vi "test.vi"() -> ()   [LabVIEW 2017]
uses:
  <vilib>/imath/engines/lvmath/Plug In/_Char/NIMS_CH_character datatype.ctl
  <vilib>/imath/engines/lvmath2/RunTimeEngine/Managers/WorkSpace/UID Generator.vi
  <vilib>/imath/engines/lvmath/Plug In/_Char/NIMS_CH_Character RV to String.vi
  <vilib>/imath/engines/lvmath2/RunTimeEngine/BuiltInFunctions/title/NIMS_title.vi
  <vilib>/imathl/engines/lvmath/Functions/Error Handling/Create Error.vi
  <vilib>/imath/engines/lvmath2/RunTimeEngine/BuiltInFunctions/xlimit/NIMS_xlimit.vi
  <vilib>/imath/engines/lvmath2/RunTimeEngine/BuiltInFunctions/ylimit/NIMS_ylimit.vi
  <vilib>/imath/engines/lvmath2/RunTimeEngine/BuiltInFunctions/hold/NIMS_hold(Enums).vi
  <vilib>/imath/engines/lvmath2/RunTimeEngine/IndexRead/NIMS M($,S).vi
  <instcachedir>/0/NIMS M($,S)_3E5749BBB62E49528D4765A77F1F6D98.lvgen/NIMS M($,S)_3E5749BBB62E49528D4765A77F1F6D98_002.vi
  <vilib>/imath/engines/lvmath2/RunTimeEngine/ErrorHandling/NIMS_Create Error From Enums.vi
  <vilib>/imath/engines/lvmath2/RunTimeEngine/BuiltInFunctions/plot/NIMS_plot(RM, RM, Str).vi
  <vilib>/imath/engines/lvmath2/RunTimeEngine/ErrorHandling/NIMS_Finalize Error.vi
  <vilib>/Utility/file.llb/Write Delimited Spreadsheet (DBL).vi
  <vilib>/vision/NI_Vision_Development_Module.lvlib
panel:
  out "robot  arrived":bool
  in  "SHOW TARGET POSITION":bool
  out "Image Out 4":T1(plugin-control)
  in  "see obstacle":bool
  out "Image Out 3":T1(plugin-control)
  in  "target array":dbl[][](array[numeric])
  out "target y position":sgl
  out "target x position":sgl
  out "robot y  position":sgl
  out "robot x position":sgl
  in  "Showing motion path":bool
  in  "robot array":dbl[][](array[numeric])
  out "robot is not in the picture":bool
  in  "check that robot is in the picture or not":bool
  out "Distance":sgl
  out "red":sgl[](array[numeric])
  out "target":sgl[](array[numeric])
  out "red Position":cluster{"x":sgl, "y":sgl}
  out "Image Out 2":T1(plugin-control)
  out "Blue Position":cluster{"x":sgl, "y":sgl}
  in  "Stop (F)":bool
  out "Image Out":T1(plugin-control)
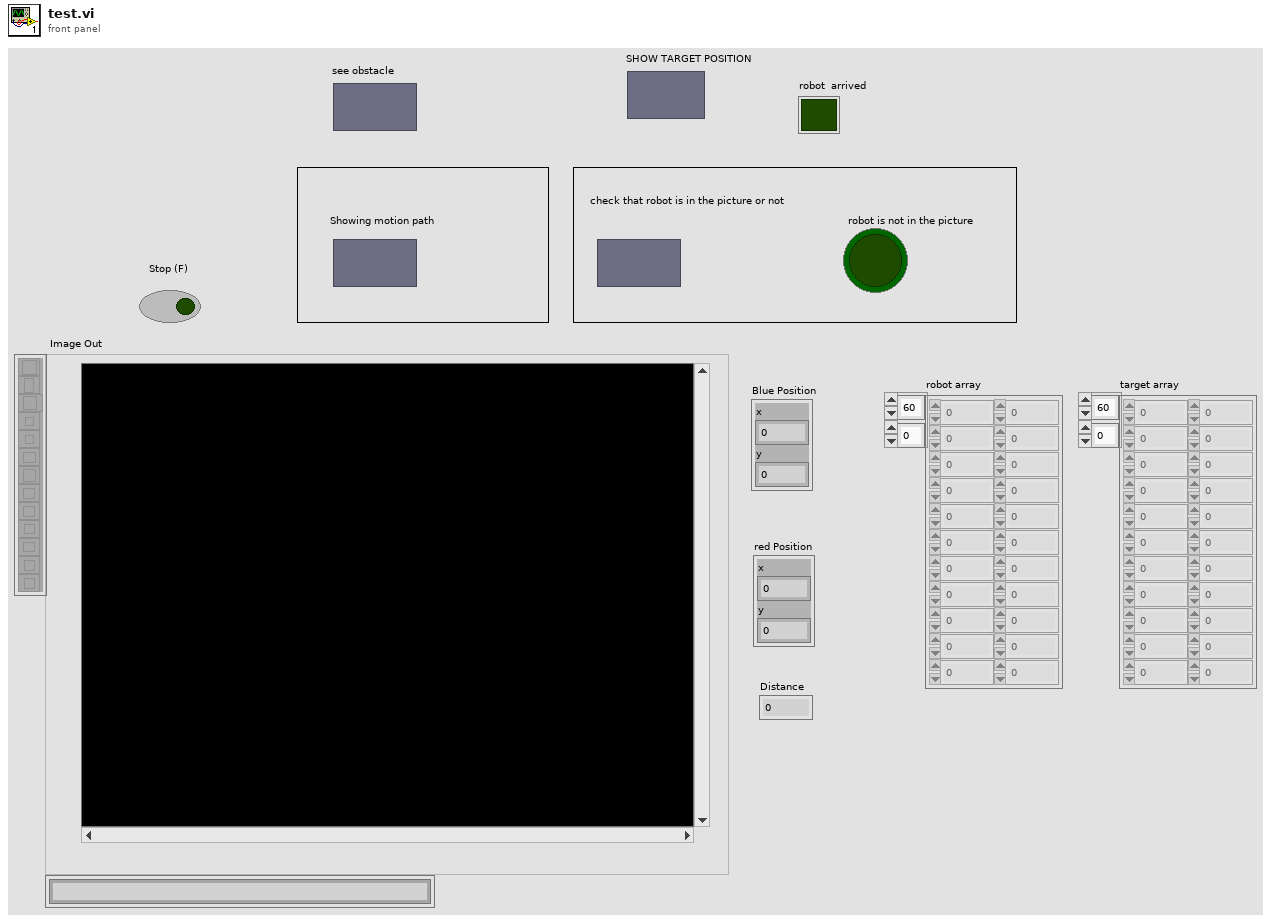
[diagram p1: front panel]
types:
  T1 = typedef "IMAQ Image.ctl" = refnum<image>
  T2 = typedef "Image Type" = u32
  T3 = typedef "NIMS_CH_character datatype.ctl" = cluster{"Numeric":u8}
  T4 = cluster{"Position":cluster{"x":sgl, "y":sgl}, "Angle":sgl, "Scale":sgl, "Score":sgl, "Bounding Box":cluster{"x":sgl, "y":sgl}[]}[]
  T5 = cluster{"Matches (Color Location 3)[0]":cluster{"Position":cluster{"x":sgl, "y":sgl}, "Angle":sgl, "Scale":sgl, "Score":sgl, "Bounding Box":cluster{"x":sgl, "y":sgl}[]}, "Matches (Color Location 3)[1]":cluster{"Position":cluster{"x":sgl, "y":sgl}, "Angle":sgl, "Scale":sgl, "Score":sgl, "Bounding Box":cluster{"x":sgl, "y":sgl}[]}, "Matches (Color Location 3)[2]":cluster{"Position":cluster{"x":sgl, "y":sgl}, "Angle":sgl, "Scale":sgl, "Score":sgl, "Bounding Box":cluster{"x":sgl, "y":sgl}[]}, "Matches (Color Location 3)[3]":cluster{"Position":cluster{"x":sgl, "y":sgl}, "Angle":sgl, "Scale":sgl, "Score":sgl, "Bounding Box":cluster{"x":sgl, "y":sgl}[]}, "Matches (Color Location 3)[4]":cluster{"Position":cluster{"x":sgl, "y":sgl}, "Angle":sgl, "Scale":sgl, "Score":sgl, "Bounding Box":cluster{"x":sgl, "y":sgl}[]}, "Matches (Color Location 3)[5]":cluster{"Position":cluster{"x":sgl, "y":sgl}, "Angle":sgl, "Scale":sgl, "Score":sgl, "Bounding Box":cluster{"x":sgl, "y":sgl}[]}, "Matches (Color Location 3)[6]":cluster{"Position":cluster{"x":sgl, "y":sgl}, "Angle":sgl, "Scale":sgl, "Score":sgl, "Bounding Box":cluster{"x":sgl, "y":sgl}[]}, "Matches (Color Location 3)[7]":cluster{"Position":cluster{"x":sgl, "y":sgl}, "Angle":sgl, "Scale":sgl, "Score":sgl, "Bounding Box":cluster{"x":sgl, "y":sgl}[]}, "Matches (Color Location 3)[8]":cluster{"Position":cluster{"x":sgl, "y":sgl}, "Angle":sgl, "Scale":sgl, "Score":sgl, "Bounding Box":cluster{"x":sgl, "y":sgl}[]}}
  T6 = cluster{"Bounding Box[0]":cluster{"x":sgl, "y":sgl}, "Bounding Box[1]":cluster{"x":sgl, "y":sgl}, "Bounding Box[2]":cluster{"x":sgl, "y":sgl}, "Bounding Box[3]":cluster{"x":sgl, "y":sgl}, "Bounding Box[4]":cluster{"x":sgl, "y":sgl}, "Bounding Box[5]":cluster{"x":sgl, "y":sgl}, "Bounding Box[6]":cluster{"x":sgl, "y":sgl}, "Bounding Box[7]":cluster{"x":sgl, "y":sgl}, "Bounding Box[8]":cluster{"x":sgl, "y":sgl}}
  T7 = cluster{"[0]":sgl, "[1]":sgl, "[2]":sgl, "[3]":sgl}
  T8 = cluster{"Matches (Color Location 1)[0]":cluster{"Position":cluster{"x":sgl, "y":sgl}, "Angle":sgl, "Scale":sgl, "Score":sgl, "Bounding Box":cluster{"x":sgl, "y":sgl}[]}, "Matches (Color Location 1)[1]":cluster{"Position":cluster{"x":sgl, "y":sgl}, "Angle":sgl, "Scale":sgl, "Score":sgl, "Bounding Box":cluster{"x":sgl, "y":sgl}[]}, "Matches (Color Location 1)[2]":cluster{"Position":cluster{"x":sgl, "y":sgl}, "Angle":sgl, "Scale":sgl, "Score":sgl, "Bounding Box":cluster{"x":sgl, "y":sgl}[]}, "Matches (Color Location 1)[3]":cluster{"Position":cluster{"x":sgl, "y":sgl}, "Angle":sgl, "Scale":sgl, "Score":sgl, "Bounding Box":cluster{"x":sgl, "y":sgl}[]}, "Matches (Color Location 1)[4]":cluster{"Position":cluster{"x":sgl, "y":sgl}, "Angle":sgl, "Scale":sgl, "Score":sgl, "Bounding Box":cluster{"x":sgl, "y":sgl}[]}, "Matches (Color Location 1)[5]":cluster{"Position":cluster{"x":sgl, "y":sgl}, "Angle":sgl, "Scale":sgl, "Score":sgl, "Bounding Box":cluster{"x":sgl, "y":sgl}[]}, "Matches (Color Location 1)[6]":cluster{"Position":cluster{"x":sgl, "y":sgl}, "Angle":sgl, "Scale":sgl, "Score":sgl, "Bounding Box":cluster{"x":sgl, "y":sgl}[]}, "Matches (Color Location 1)[7]":cluster{"Position":cluster{"x":sgl, "y":sgl}, "Angle":sgl, "Scale":sgl, "Score":sgl, "Bounding Box":cluster{"x":sgl, "y":sgl}[]}, "Matches (Color Location 1)[8]":cluster{"Position":cluster{"x":sgl, "y":sgl}, "Angle":sgl, "Scale":sgl, "Score":sgl, "Bounding Box":cluster{"x":sgl, "y":sgl}[]}}
  T9 = cluster{"Matches (Color Location 2)[0]":cluster{"Position":cluster{"x":sgl, "y":sgl}, "Angle":sgl, "Scale":sgl, "Score":sgl, "Bounding Box":cluster{"x":sgl, "y":sgl}[]}, "Matches (Color Location 2)[1]":cluster{"Position":cluster{"x":sgl, "y":sgl}, "Angle":sgl, "Scale":sgl, "Score":sgl, "Bounding Box":cluster{"x":sgl, "y":sgl}[]}, "Matches (Color Location 2)[2]":cluster{"Position":cluster{"x":sgl, "y":sgl}, "Angle":sgl, "Scale":sgl, "Score":sgl, "Bounding Box":cluster{"x":sgl, "y":sgl}[]}, "Matches (Color Location 2)[3]":cluster{"Position":cluster{"x":sgl, "y":sgl}, "Angle":sgl, "Scale":sgl, "Score":sgl, "Bounding Box":cluster{"x":sgl, "y":sgl}[]}, "Matches (Color Location 2)[4]":cluster{"Position":cluster{"x":sgl, "y":sgl}, "Angle":sgl, "Scale":sgl, "Score":sgl, "Bounding Box":cluster{"x":sgl, "y":sgl}[]}, "Matches (Color Location 2)[5]":cluster{"Position":cluster{"x":sgl, "y":sgl}, "Angle":sgl, "Scale":sgl, "Score":sgl, "Bounding Box":cluster{"x":sgl, "y":sgl}[]}, "Matches (Color Location 2)[6]":cluster{"Position":cluster{"x":sgl, "y":sgl}, "Angle":sgl, "Scale":sgl, "Score":sgl, "Bounding Box":cluster{"x":sgl, "y":sgl}[]}, "Matches (Color Location 2)[7]":cluster{"Position":cluster{"x":sgl, "y":sgl}, "Angle":sgl, "Scale":sgl, "Score":sgl, "Bounding Box":cluster{"x":sgl, "y":sgl}[]}, "Matches (Color Location 2)[8]":cluster{"Position":cluster{"x":sgl, "y":sgl}, "Angle":sgl, "Scale":sgl, "Score":sgl, "Bounding Box":cluster{"x":sgl, "y":sgl}[]}}
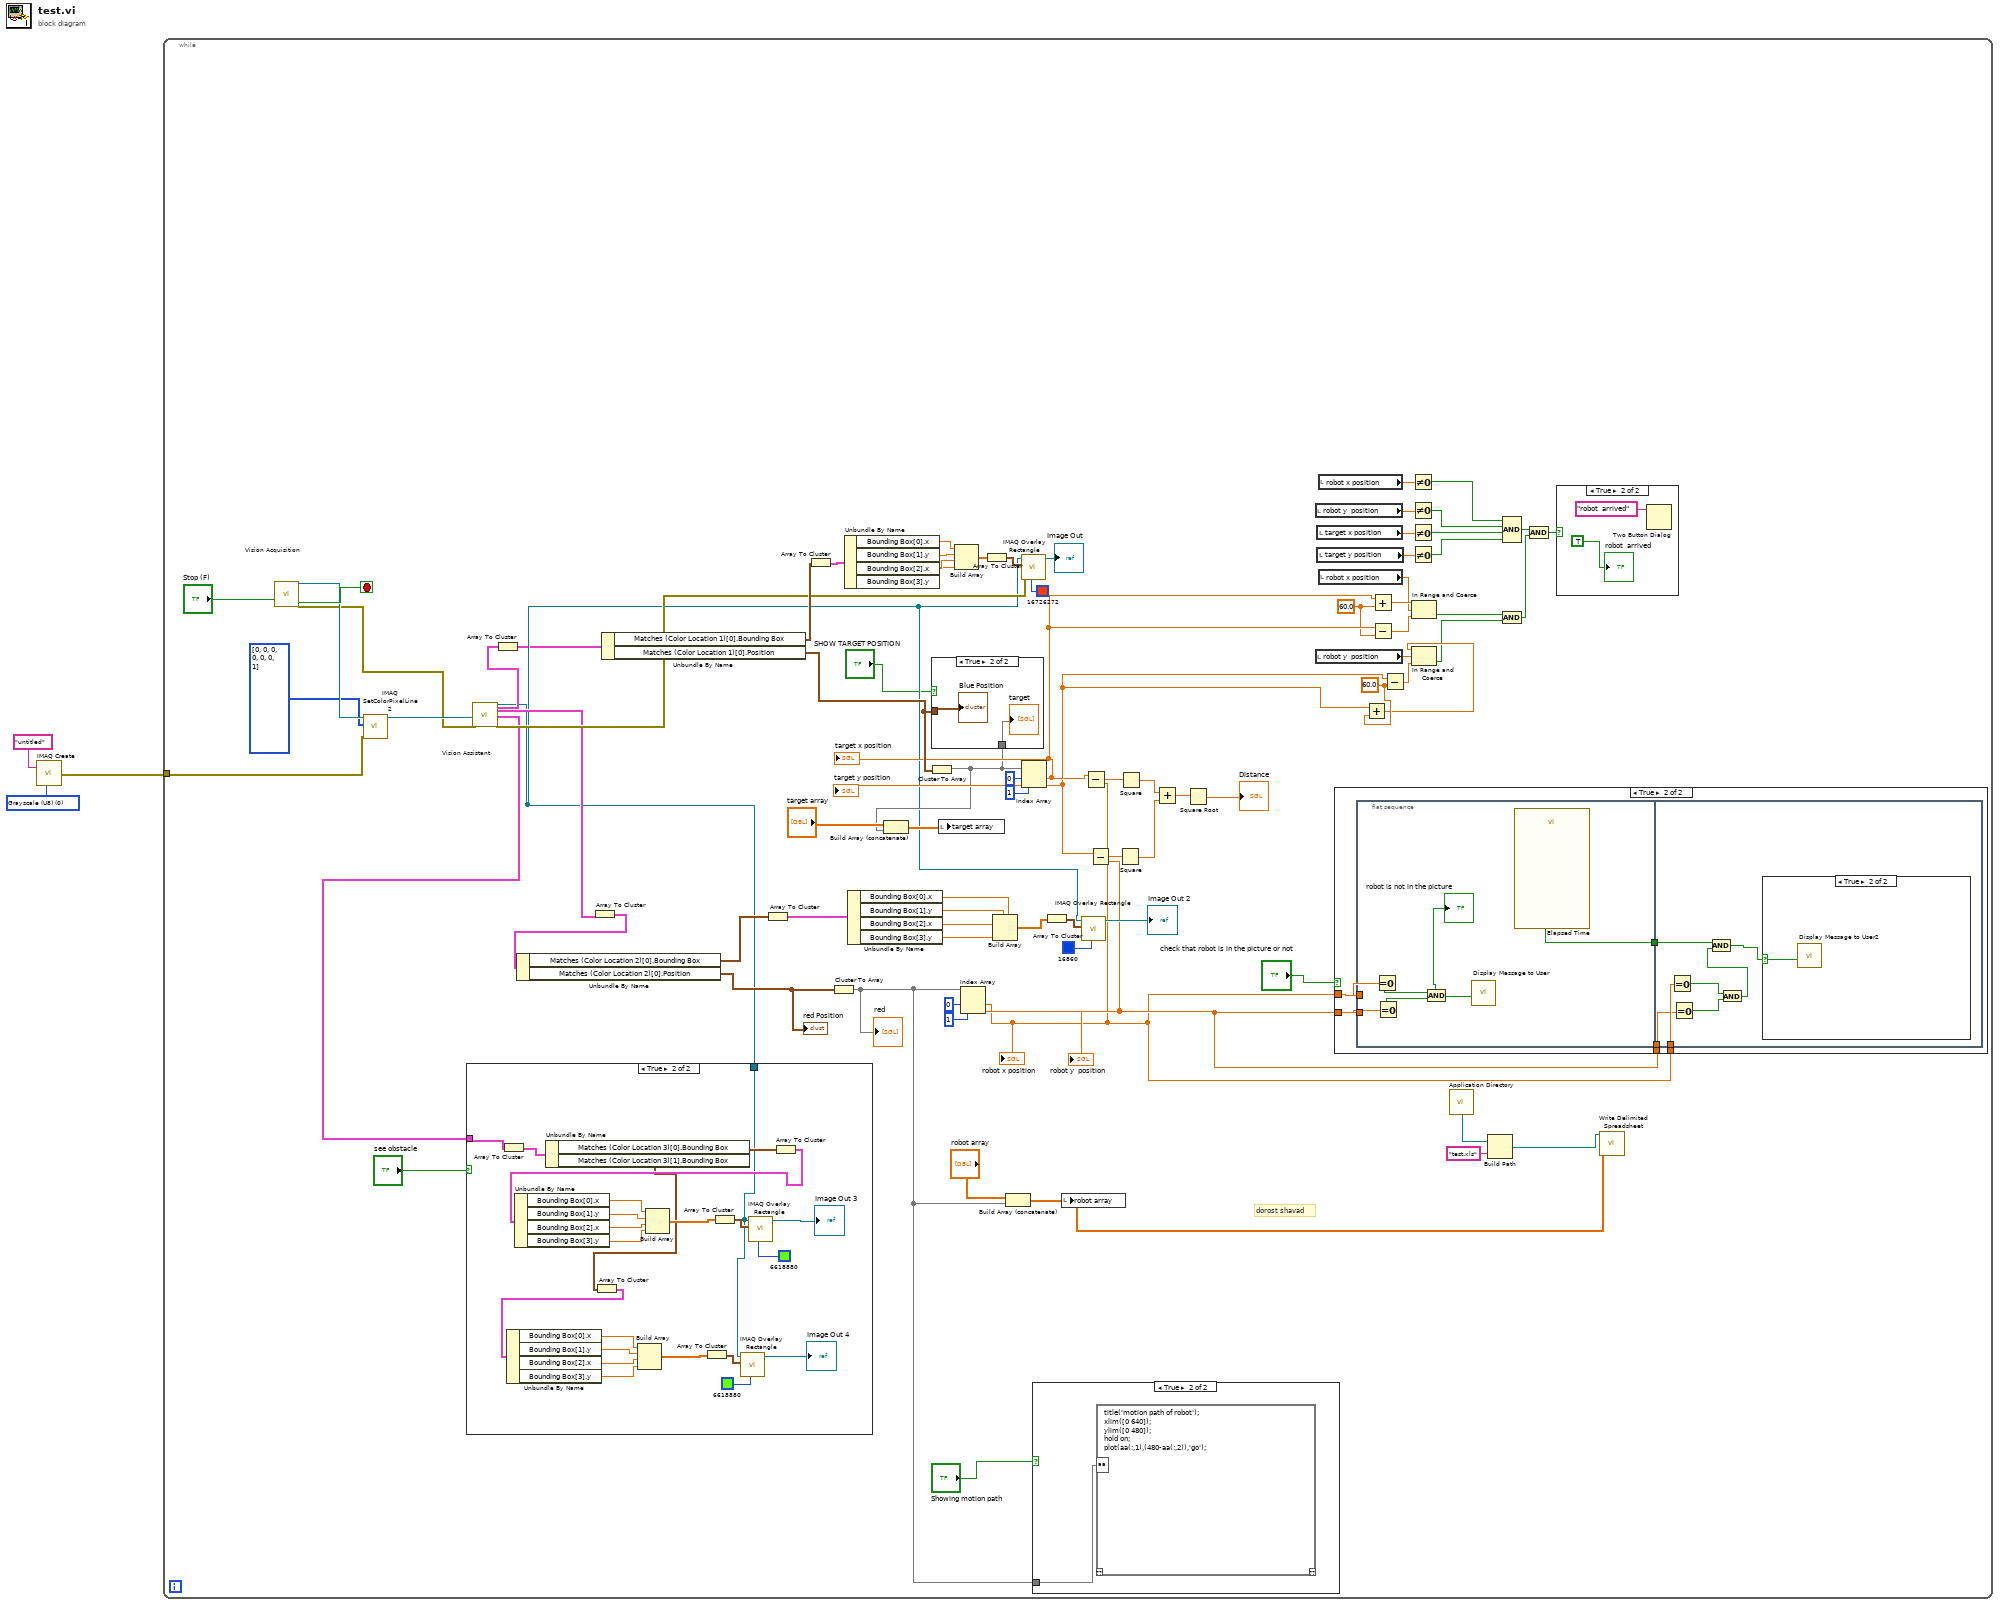
[diagram p0: block diagram]
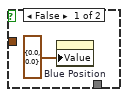
[diagram p2: hidden frame]
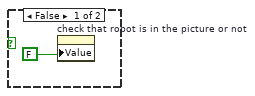
[diagram p7: hidden frame]
diagram:
  w2 = T2 0 items=["Grayscale (U8)", "Grayscale (I16)", "Grayscale (SGL)", "Complex (CSG)", "RGB (U32)", "HSL (U32)", "RGB (U64)", "Grayscale (U16)"] ("Image Type")
  n1 = call "IMAQ Create"("Image Name"="untitled", "Image Type"=w2) -> ("error out"=w1:errorcluster)  [unwired: 3 in, 1 out]
  n2 = while {
    tunnel: w1 -> [w84]
    stop <- w86 stop-if-true
    w30 = 60.0
    w32 = 60.0
    # "dorost shavad"
    n3 = call "Vision Acquisition"("Stop (F)"="Stop (F)") -> ("Image Out"=w85:T1, "Stopped"=w86:bool, "error out"=w55:errorcluster)  [unwired: 24 in]
    n4 = call "IMAQ SetColorPixelLine 2"("error in (no error)"=w84, "Line Coordinates"=i32[] [0, 0, 0, 0, 0, 0, 1], "Image"=w85) -> ("Image Out"=w56:T1)  [unwired: 7 in, 1 out]
    n5 = call "Vision Assistant"("Image In"=w56, "error in"=w55) -> ("Image Out"=w8:T1, "Matches (Color Location 1)"=w53:T4, "Matches (Color Location 2)"=w52:T4, "Matches (Color Location 3)"=w9:T4, "error out"=w54:errorcluster)  [unwired: 20 in, 1 out]
    n6 = case shown="True" "see obstacle" {
      tunnel: w9 -> [_ w113]
      tunnel: w8 -> [_ w91]
      frame False {
      }
      frame True {
        n7 = Array To Cluster(array=w113) -> (cluster=w112:T5)
        n8 = Unbundle By Name(w112) -> ("Matches (Color Location 3)[0].Bounding Box"=w111:cluster{"x":sgl, "y":sgl}[], "Matches (Color Location 3)[1].Bounding Box"=w93:cluster{"x":sgl, "y":sgl}[])
        n9 = Array To Cluster(array=w93) -> (cluster=w92:T6)
        n10 = Unbundle By Name(w92) -> ("Bounding Box[0].x"=w98:sgl, "Bounding Box[1].y"=w97:sgl, "Bounding Box[2].x"=w96:sgl, "Bounding Box[3].y"=w95:sgl)
        n11 = Build Array(w98, w97, w96, w95) -> (w99:sgl[])
        n12 = Array To Cluster(array=w99) -> (cluster=w100:T7)
        n13 = call "IMAQ Overlay Rectangle"("Color"=u32 6618880, "Rectangle"=w100, "Image"=w91) -> ("Image Out"=→"Image Out 4":T1)  [unwired: 7 in, 1 out]
        n14 = Array To Cluster(array=w111) -> (cluster=w110:T6)
        n15 = Unbundle By Name(w110) -> ("Bounding Box[0].x"=w106:sgl, "Bounding Box[1].y"=w105:sgl, "Bounding Box[2].x"=w104:sgl, "Bounding Box[3].y"=w103:sgl)
        n16 = Build Array(w106, w105, w104, w103) -> (w107:sgl[])
        n17 = Array To Cluster(array=w107) -> (cluster=w108:T7)
        n18 = call "IMAQ Overlay Rectangle"("Color"=u32 6618880, "Rectangle"=w108, "Image"=w91) -> ("Image Out"=→"Image Out 3":T1)  [unwired: 7 in, 1 out]
      }
    }
    n19 = Array To Cluster(array=w53) -> (cluster=w5:T8)
    n20 = Array To Cluster(array=w52) -> (cluster=w51:T9)
    n21 = Unbundle By Name(w51) -> ("Matches (Color Location 2)[0].Bounding Box"=w46:cluster{"x":sgl, "y":sgl}[], "Matches (Color Location 2)[0].Position"=w45:cluster{"x":sgl, "y":sgl})
    "red Position" <- w45
    n22 = Unbundle By Name(w5) -> ("Matches (Color Location 1)[0].Bounding Box"=w83:cluster{"x":sgl, "y":sgl}[], "Matches (Color Location 1)[0].Position"=w67:cluster{"x":sgl, "y":sgl})
    n23 = Array To Cluster(array=w46) -> (cluster=w74:T6)
    n24 = Array To Cluster(array=w83) -> (cluster=w82:T6)
    n25 = Cluster To Array(cluster=w45) -> (array=w39:sgl[])
    "red" <- w39
    n26 = Unbundle By Name(w82) -> ("Bounding Box[0].x"=w81:sgl, "Bounding Box[1].y"=w80:sgl, "Bounding Box[2].x"=w79:sgl, "Bounding Box[3].y"=w78:sgl)
    n27 = Unbundle By Name(w74) -> ("Bounding Box[0].x"=w73:sgl, "Bounding Box[1].y"=w72:sgl, "Bounding Box[2].x"=w71:sgl, "Bounding Box[3].y"=w70:sgl)
    n28 = Cluster To Array(cluster=w67) -> (array=w11:sgl[])
    n29 = Build Array (concatenate)("target array", w11) -> (w10:dbl[][])
    n30 = case shown="True" "SHOW TARGET POSITION" {
      tunnel: w67 -> [_ w90]
      tunnel: w11 -> [_ w89]
      frame False {
        n31 = property on="Blue Position" class="Clust (strict)"("Value"=cluster{"x":sgl, "y":sgl} {"x"=0.0, "y"=0.0} ("Blue Position")) -> ()  [unwired: 2 in, 2 out]
      }
      frame True {
        "Blue Position" <- w90
        "target" <- w89
      }
    }
    n32 = local write "target array"(w10) -> ()
    n33 = Build Array(w81, w80, w79, w78) -> (w77:sgl[])
    n34 = Index Array(array=w39, index #1=0 ("index"), index #2=1 ("index")) -> (element #1=w41:sgl, element #2=w49:sgl)
    "robot x position" <- w41
    "robot y  position" <- w49
    n35 = Array To Cluster(array=w77) -> (cluster=w75:T7)
    n36 = Build Array(w73, w72, w71, w70) -> (w42:sgl[])
    n37 = Build Array (concatenate)("robot array", w39) -> (w4:dbl[][])
    n38 = call "IMAQ Overlay Rectangle"("Color"=u32 16726272, "error in (no error)"=w54, "Rectangle"=w75, "Image"=w8) -> ("Image Out"=→"Image Out":T1)  [unwired: 6 in, 1 out]
    n39 = Index Array(array=w11, index #1=0 ("index"), index #2=1 ("index")) -> (element #1=w33:sgl, element #2=w31:sgl)
    "target x position" <- w33
    "target y position" <- w31
    n40 = case shown="True" "Showing motion path" {
      tunnel: w39 -> [_ w116]
      frame False {
      }
      frame True {
        n41 = mathscript code="title('motion path of robot');\nxlim([0 640]);\nylim([0 480]);\nhold on;\nplot(aa(:,1),(480-aa(:,2)),'go');"("aa"=w116) -> ()  [unwired: 1 in, 1 out]
      }
    }
    n42 = Array To Cluster(array=w42) -> (cluster=w68:T7)
    n43 = local write "robot array"(w4) -> ()
    n44 = call "IMAQ Overlay Rectangle"("Color"=u32 16860, "Rectangle"=w68, "Image"=w8) -> ("Image Out"=→"Image Out 2":T1)  [unwired: 7 in, 1 out]
    n45 = Subtract(x=w33, y=w41) -> (x-y=w62:sgl)
    n46 = Subtract(x=w31, y=w49) -> (x-y=w61:sgl)
    n47 = Square(x=w61) -> (x^2=w59:sgl)
    n48 = Square(x=w62) -> (x^2=w60:sgl)
    n49 = Add(x=w60, y=w59) -> (x+y=w58:sgl)
    n50 = Square Root(x=w58) -> (sqrt(x)=→"Distance":sgl)
    n51 = local read "robot y  position"() -> (w23:sgl)
    n52 = local read "robot y  position"() -> (w27:sgl)
    n53 = local read "target x position"() -> (w22:sgl)
    n54 = local read "target y position"() -> (w21:sgl)
    n55 = local read "robot x position"() -> (w24:sgl)
    n56 = local read "robot x position"() -> (w34:sgl)
    n57 = case shown="True" "check that robot is in the picture or not" {
      tunnel: w49 -> [_ w247]
      tunnel: w41 -> [_ w246]
      tunnel: w41 -> [_ w245]
      tunnel: w49 -> [_ w244]
      frame False {
      }
      frame True {
        n58 = flat-sequence {
          tunnel: w247 -> [w251]
          tunnel: w246 -> [w250]
          tunnel: [w248] -> w243
          tunnel: w245 -> [w258]
          tunnel: w244 -> [w257]
          tunnel: w243 -> [w254]
          frame #0 {
            n59 = Equal To 0?(x=w250) -> (x = 0?=w252:bool)
            n60 = Equal To 0?(x=w251) -> (x = 0?=w253:bool)
            n61 = And(x=w252, y=w253) -> (x .and. y?=w249:bool)
            "robot is not in the picture" <- w249
            n62 = call "Display Message to User"("Enable"=w249) -> ()  [unwired: 9 in, 2 out]
            n63 = call "Elapsed Time"() -> ("Time has Elapsed"=w248:bool)  [unwired: 12 in, 7 out]
          }
          frame #1 {
            n64 = Equal To 0?(x=w258) -> (x = 0?=w259:bool)
            n65 = Equal To 0?(x=w257) -> (x = 0?=w260:bool)
            n66 = And(x=w259, y=w260) -> (x .and. y?=w255:bool)
            n67 = And(x=w254, y=w255) -> (x .and. y?=w256:bool)
            n68 = case shown="True" w256 {
              selector: w256 -> [_ w262]
              frame False {
                n69 = property on="check that robot is in the picture or not" class="Bool (strict)"("Value"=FALSE) -> ()  [unwired: 2 in, 2 out]
              }
              frame True {
                n70 = call "Display Message to User2"("Enable"=w262) -> ()  [unwired: 9 in, 2 out]
              }
            }
          }
        }
      }
    }
    n71 = Add(x=w31, y=w30) -> (x+y=w29:dbl)
    n72 = Add(x=w33, y=w32) -> (x+y=w36:dbl)
    n73 = Subtract(x=w33, y=w32) -> (x-y=w35:dbl)
    n74 = Subtract(x=w31, y=w30) -> (x-y=w28:dbl)
    n75 = Not Equal To 0?(x=w24) -> (x != 0?=w20:bool)
    n76 = Not Equal To 0?(x=w23) -> (x != 0?=w19:bool)
    n77 = Not Equal To 0?(x=w22) -> (x != 0?=w18:bool)
    n78 = Not Equal To 0?(x=w21) -> (x != 0?=w17:bool)
    n79 = In Range and Coerce(upper limit=w36, x=w34, lower limit=w35) -> (In Range?=w26:bool)  [unwired: 1 out]
    n80 = In Range and Coerce(upper limit=w29, x=w27, lower limit=w28) -> (In Range?=w25:bool)  [unwired: 1 out]
    n81 = call <vilib>:"Application Directory.vi"() -> ("Application Directory"=w38:path)
    n82 = Build Path(base path=w38, name or relative path="test.xls") -> (appended path=w13:path)
    n83 = And(x=w26, y=w25) -> (x .and. y?=w16:bool)
    n84 = Compound Arithmetic op=AND(w20, w19, w18, w17) -> (w15:bool)
    n85 = And(x=w15, y=w16) -> (x .and. y?=w14:bool)
    n86 = case shown="True" w14 {
      frame False {
      }
      frame True {
        n87 = Two Button Dialog(message="robot  arrived") -> ()  [unwired: 2 in, 1 out]
        "robot  arrived" <- TRUE
      }
    }
    n88 = call-poly <vilib>:"Write Delimited Spreadsheet.vi"("file path (dialog if empty)"=w13, "2D data"=w4) -> ()  [unwired: 12 in, 2 out]
  }
